vi "DEMO AC.vi"(10 "SectionProperties":T1, 11 "AC Config":T4={"Board 1 alias"="AO-1/ao0:31", "Board 1 Enable"=TRUE, "Board 2 alias"="AO-2/ao0:31", "Board 2 Enable"=TRUE}) -> (0 "error out":errorcluster)   [LabVIEW 2019, in "ArrayController.lvclass"]
uses:
  ArrayController.lvclass
  ACConfig.ctl
  Datalog/DatalogSubvis/SearchableTag.ctl
  Sequence/SequenceSubvis/RF Direction.ctl
  Sequence/SequenceSubvis/PolarizationSelect.ctl
  Datalog/DataLog.lvclass
panel:
  in  "stop":bool
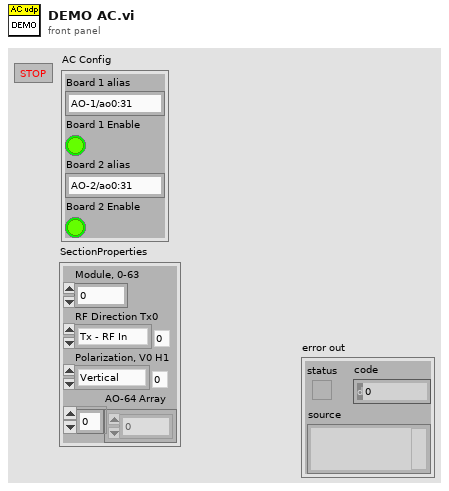
[diagram p1: front panel]
types:
  T1 = typedef "DataLog.lvclass/SearchableTag.ctl" = cluster{"Module, 0-63":i32, "RF Direction Tx0":T2, "Polarization, V0 H1":T3, "AO-64 Array":dbl[]}
  T2 = typedef "RF Direction.ctl" = enum16{"Tx - RF In", "Rx - RF Out"}
  T3 = typedef "PolarizationSelect.ctl" = enum16{"Vertical", "Horizontal"}
  T4 = typedef "ACConfig.ctl" = cluster{"Board 1 alias":string, "Board 1 Enable":bool, "Board 2 alias":string, "Board 2 Enable":bool}
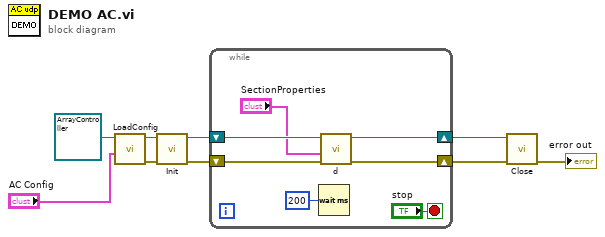
[diagram p0: block diagram]
diagram:
  n1 = call "LoadConfig.vi"("AC Config"="AC Config", "ArrayController in"=refnum<class "ArrayController.lvclass"> refnum) -> ("error out"=w3:errorcluster, "ArrayController out"=w5:refnum<class "ArrayController.lvclass">)  [unwired: 8 in]
  n2 = call "Init.vi"("error in (no error)"=w3, "ArrayController in"=w5) -> ("error out"=w6:errorcluster, "ArrayController out"=w7:refnum<class "ArrayController.lvclass">)  [unwired: 8 in]
  n3 = while {
    shift-right: [w13] -> w2
    shift-left: w7 -> [w16]
    shift-right: [w12] -> w1
    shift-left: w6 -> [w15]
    stop <- "stop" stop-if-true
    n4 = Wait (ms)(milliseconds to wait=u32 200) -> ()  [unwired: 1 out]
    n5 = call "d.vi"("error in (no error)"=w15, "d Cmd Properties"="SectionProperties", "ArrayController in"=w16) -> ("error out"=w12:errorcluster, "ArrayController out"=w13:refnum<class "ArrayController.lvclass">)  [unwired: 7 in]
  }
  n6 = call "Close.vi"("error in (no error)"=w1, "ArrayController in"=w2) -> ("error out"=→"error out":errorcluster)  [unwired: 8 in, 1 out]
